vi "Run.vi"(7 "Team Index":i32, 8 "Column":i32, 9 "Row":i32, 10 "View":i32[](array[numeric]) caption="View (Team Index, -1: empty)", 11 "Assassin In":refnum<class "Assassin.lvclass">) -> (0 "Replicated":refnum<class "Square.lvclass">, 1 "Direction":T1, 2 "Action":T2, 3 "Square Out":refnum<class "Square.lvclass">)   [LabVIEW 2015, in "Assassin.lvclass"]
uses:
  Assassin.lvclass
  Square/Square.lvclass
  Type Defs/Action Enum.ctl
  Type Defs/Direction Enum.ctl
  Common/Position.ctl
  Assassin.lvclass/Assassin.ctl
  SubVIs/Read-Only Globals.vi
  SubVIs/Globals (private).vi
  Common/Find Enemy.vi
  Common/Reverse Direction.vi
  SubVIs/Read-Only Stats.vi
  Common/Common.lvlib
  Type Defs/SB Type Defs.lvlib
panel:
  # "NW\nN\nNE\nE\nSE\nS\nSW\nW"
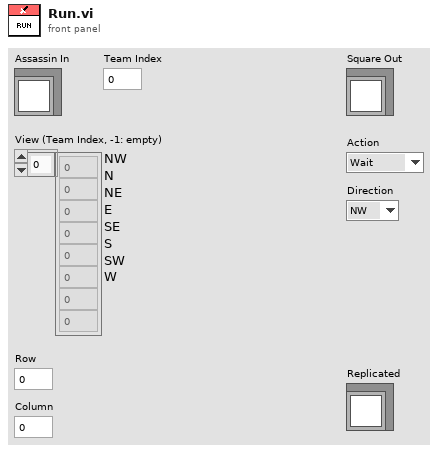
[diagram p1: front panel]
types:
  T1 = typedef "SB Type Defs.lvlib/Direction Enum.ctl" = enum16{"NW", "N", "NE", "E", "SE", "S", "SW", "W"}
  T2 = typedef "SB Type Defs.lvlib/Action Enum.ctl" = enum16{"Wait", "Move", "Attack", "Replicate"}
  T3 = typedef "Common.lvlib/Position.ctl" = cluster{"Column":i32, "Row":i32}
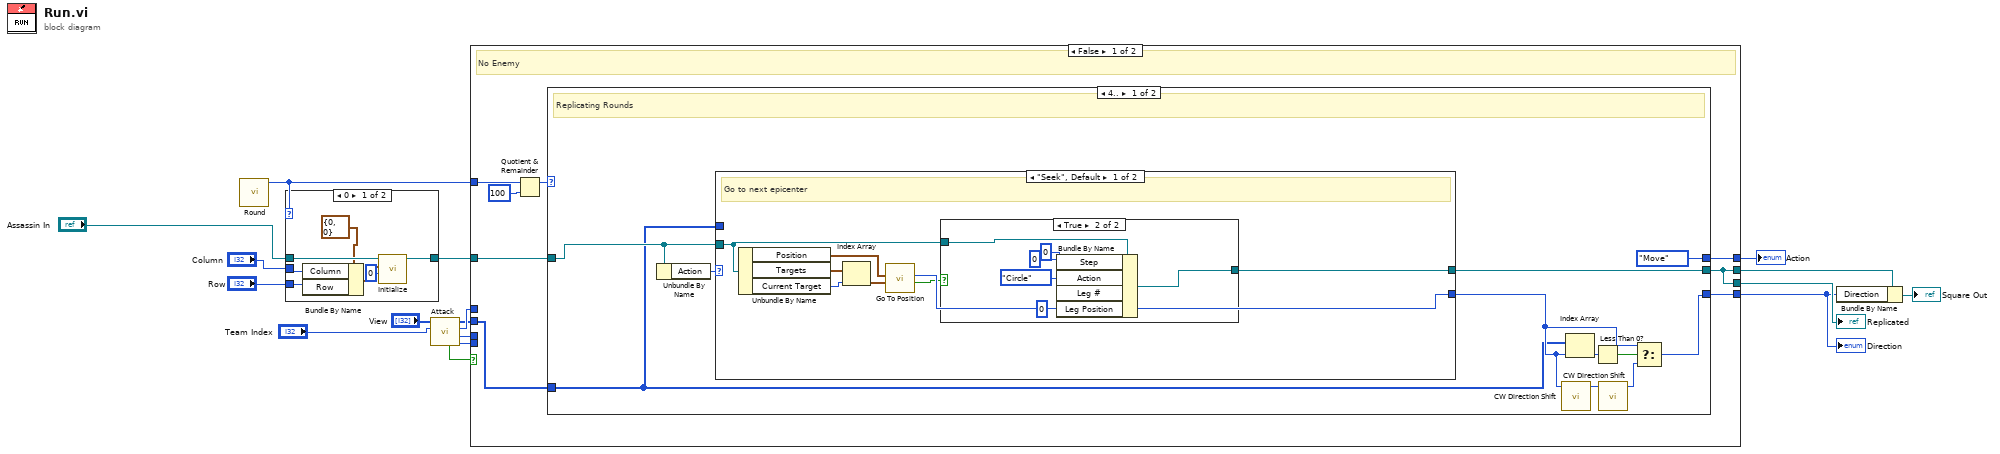
[diagram p0: block diagram]
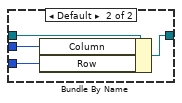
[diagram p2: hidden frame]
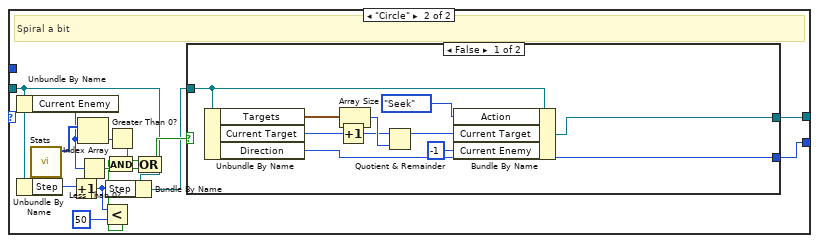
[diagram p4: hidden frame]
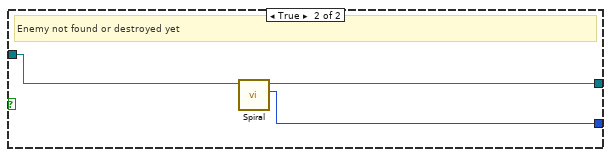
[diagram p5: hidden frame]
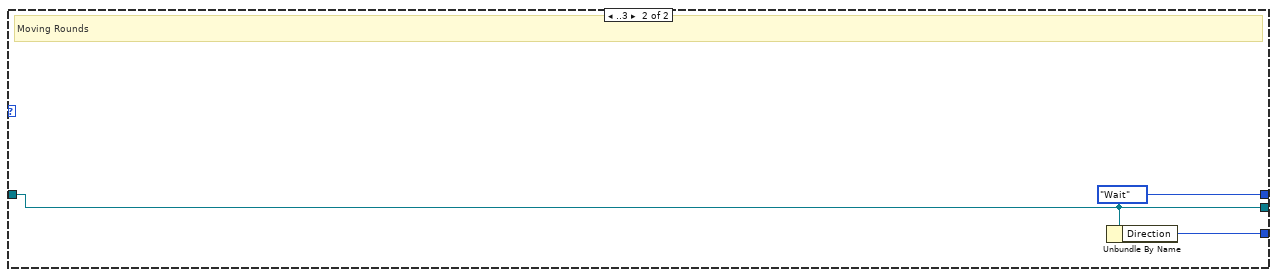
[diagram p6: hidden frame]
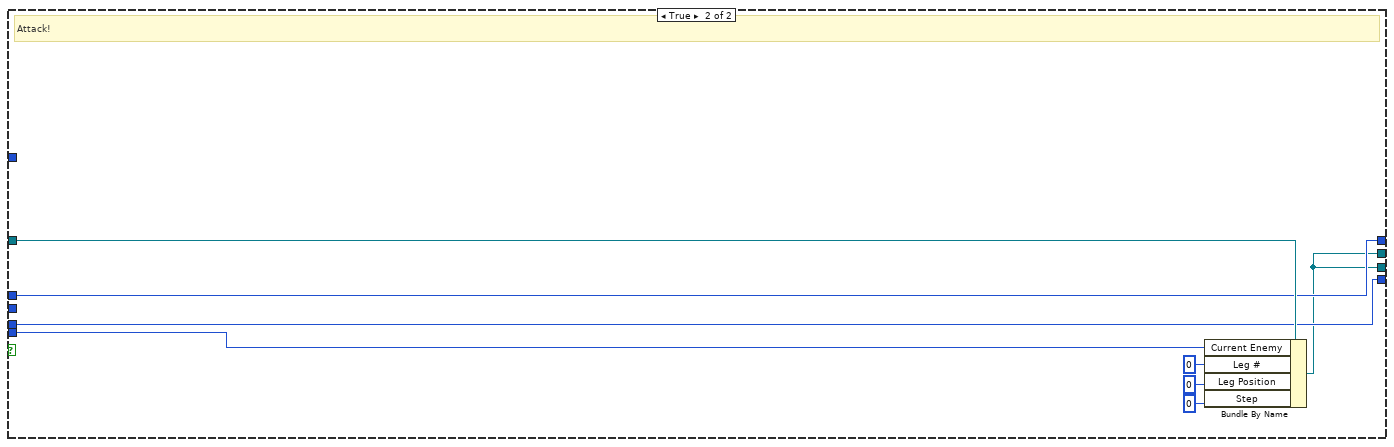
[diagram p7: hidden frame]
diagram:
  n1 = call "Round.vi"() -> ("Round"=w1:i32)  [unwired: 11 in]
  n2 = case shown="0" w1 {
    tunnel: "Assassin In" -> [w24 w28]
    tunnel: [w23 w27] -> w9
    tunnel: "Column" -> [w20 w26]
    tunnel: "Row" -> [w19 w25]
    frame 0 {
      n3 = Bundle By Name(cluster=T3 {"Column"=0, "Row"=0} ("Position"), "Column"=w20, "Row"=w19) -> (w21:T3)
      n4 = call "Initialize.vi"("Current Target"=0, "Position"=w21, "Assassin in"=w24) -> ("Assassin out"=w23:refnum<class "Assassin.lvclass">)  [unwired: 8 in]
    }
    frame Default {
      n5 = Bundle By Name(cluster=w28, "Column"=w26, "Row"=w25) -> (w27:refnum<class "Assassin.lvclass">)
    }
  }
  n6 = call "Attack.vi"("Team Index"="Team Index", "View"="View") -> ("Enemy"=w2:i32, "Direction"=w10:i32, "Action"=w11:T2, "View"=w3:i32[], "Enemy Found?"=w12:bool)  [unwired: 4 in, 1 out]
  n7 = case shown="False" w12 {
    tunnel: w9 -> [w33 w101]
    tunnel: [w34 w98] -> w15
    tunnel: [w36 w100] -> w14
    tunnel: [w35 w99] -> w7
    tunnel: [w34 w98] -> w13
    tunnel: w11 -> [_ w100]
    tunnel: w10 -> [_ w99]
    tunnel: w1 -> [w32 _]
    tunnel: w3 -> [w29 _]
    tunnel: w2 -> [_ w97]
    frame False {
      # "No Enemy"
      n8 = Quotient & Remainder(x=w32, y=100) -> (x-y*floor(x/y)=w30:i32)  [unwired: 1 out]
      n9 = case shown="4.." w30 {
        tunnel: [Action_Enum."Move" ("Action") Action_Enum."Wait" ("Action")] -> w36
        tunnel: [w42 w91] -> w35
        tunnel: [w46 w92] -> w34
        tunnel: w33 -> [w45 w92]
        tunnel: w29 -> [w37 _]
        frame 4.. {
          # "Replicating Rounds"
          n10 = Unbundle By Name(w45) -> ("Action"=w38:enum16{"Seek", "Circle"})
          n11 = case shown="\"Seek\", Default" w38 {
            tunnel: w45 -> [w52 w66]
            tunnel: [w55 w74] -> w40
            tunnel: [w53 w75] -> w46
            tunnel: w37 -> [_ _]
            frame "Seek", Default {
              # "Go to next epicenter"
              n12 = Unbundle By Name(w52) -> ("Position"=w51:T3, "Targets"=w50:T3[], "Current Target"=w48:i32)
              n13 = Index Array(array=w50, index=w48) -> (element=w49:T3)
              n14 = call "Go To Position.vi"("Target Position"=w49, "My Position"=w51) -> ("Arrived?"=w54:bool, "Direction"=w55:T1)  [unwired: 7 in, 1 out]
              n15 = case shown="True" w54 {
                tunnel: w52 -> [w56 w62]
                tunnel: [w56 w61] -> w53
                frame False {
                }
                frame True {
                  n16 = Bundle By Name(cluster=w62, "Step"=0, "Action"=enum16{"Seek", "Circle"}."Circle", "Leg #"=0, "Leg Position"=0) -> (w61:refnum<class "Assassin.lvclass">)
                }
              }
            }
            frame "Circle" {
              # "Spiral a bit"
              n17 = Unbundle By Name(w66) -> ("Current Enemy"=w73:i32)
              n18 = Unbundle By Name(w66) -> ("Step"=w67:i32)
              n19 = call "Stats.vi"() -> ("Squares"=w77:i32[])  [unwired: 7 in, 4 out]
              n20 = Increment(x=w67) -> (x+1=w68:i32)
              n21 = Index Array(array=w77, index=w73) -> (element=w76:i32)
              n22 = Less Than 0?(x=w73) -> (x < 0?=w70:bool)
              n23 = Less?(x=w68, y=50) -> (x < y?=w63:bool)
              n24 = And(x=w63, y=w70) -> (x .and. y?=w64:bool)
              n25 = Bundle By Name(cluster=w66, "Step"=w68) -> (w65:refnum<class "Assassin.lvclass">)
              n26 = Greater Than 0?(x=w76) -> (x > 0?=w72:bool)
              n27 = Compound Arithmetic op=OR(w72, w64) -> (w71:bool)
              n28 = case shown="False" w71 {
                tunnel: w65 -> [w85 w88]
                tunnel: [w86 w90] -> w75
                tunnel: [w83 w89] -> w74
                frame False {
                  n29 = Unbundle By Name(w85) -> ("Targets"=w82:T3[], "Current Target"=w84:i32, "Direction"=w83:T1)
                  n30 = Increment(x=w84) -> (x+1=w80:i32)
                  n31 = Array Size(array=w82) -> (size(s)=w81:i32)
                  n32 = Quotient & Remainder(x=w80, y=w81) -> (x-y*floor(x/y)=w79:i32)  [unwired: 1 out]
                  n33 = Bundle By Name(cluster=w85, "Action"=enum16{"Seek", "Circle"}."Seek", "Current Target"=w79, "Current Enemy"=-1) -> (w86:refnum<class "Assassin.lvclass">)
                }
                frame True {
                  # "Enemy not found or destroyed yet"
                  n34 = call "Spiral.vi"("Assassin in"=w88) -> ("Direction"=w89:T1, "output cluster"=w90:refnum<class "Assassin.lvclass">)  [unwired: 9 in]
                }
              }
            }
          }
          n35 = call "CW Direction Shift.vi"("Direction"=w40) -> ("Numeric"=w41:i32)  [unwired: 10 in]
          n36 = Index Array(array=w37, index=w40) -> (element=w44:i32)
          n37 = Less Than 0?(x=w44) -> (x < 0?=w43:bool)
          n38 = call "CW Direction Shift.vi"("Direction"=w41) -> ("Numeric"=w39:i32)  [unwired: 10 in]
          n39 = Select(t=w40, s=w43, f=w39) -> (s? t:f=w42:i32)
        }
        frame ..3 {
          # "Moving Rounds"
          n40 = Unbundle By Name(w92) -> ("Direction"=w91:T1)
        }
      }
    }
    frame True {
      # "Attack!"
      n41 = Bundle By Name(cluster=w101, "Current Enemy"=w97, "Leg #"=0, "Leg Position"=0, "Step"=0) -> (w98:refnum<class "Assassin.lvclass">)
    }
  }
  "Action" <- w14
  "Direction" <- w7
  "Replicated" <- w13
  n42 = Bundle By Name(cluster=w15, "Direction"=w7) -> (→"Square Out":refnum<class "Assassin.lvclass">)
